vi "EnqueueManualMode.vi"(6 "Priority?":bool, 8 "error in (no error)":errorcluster, 9 "Data":variant, 10 "Message":T1, 11 "queue":refnum<queue>) -> (0 "error out":errorcluster, 3 "queue out":refnum<queue>)   [LabVIEW 2019, in "ManualMode.lvlib"]
uses:
  ManualMode.lvlib
  Enum - ManualModeMessage.ctl
  Cluster - ManualModeMessageCluster.ctl
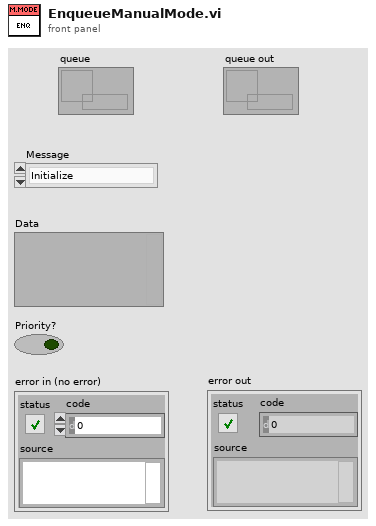
[diagram p1: front panel]
types:
  T1 = typedef "ManualMode.lvlib/Enum - ManualModeMessage.ctl" = enum16{"Initialize", "Idle", "Start", "Stop", "Pause", "Resume", "BroadcastPreCollection", "MoveCCW", "MoveCW", "StopMove", "SetZero", "GotoZero", "UpdateHW", "SendMark10Cmd", "ReadPosition", "ReadTorque", "ReadStatus", "Error", "Exit"}
  T2 = typedef "ManualMode.lvlib/Cluster - ManualModeMessageCluster.ctl" = cluster{"Message":T1, "Data":variant}
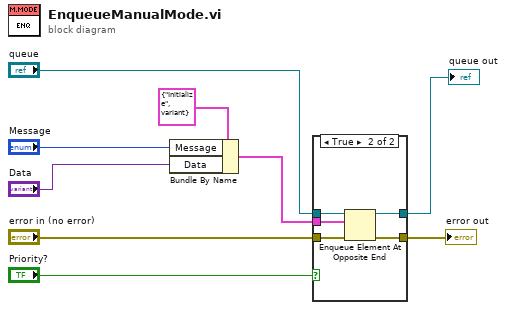
[diagram p0: block diagram]
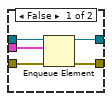
[diagram p2: hidden frame]
diagram:
  n1 = Bundle By Name(cluster=T2 {"Message"=enum."Initialize", "Data"=variant} ("element"), "Message"="Message", "Data"="Data") -> (w7:T2)
  n2 = case shown="True" "Priority?" {
    tunnel: [w14 w18] -> w9
    tunnel: w7 -> [w13 w15]
    tunnel: "queue" -> [w12 w17]
    tunnel: "error in (no error)" -> [w11 w19]
    tunnel: [w10 w16] -> w2
    frame False {
      n3 = Enqueue Element(queue=w12, element=w13, error in (no error)=w11) -> (queue out=w10:refnum<queue>, error out=w14:errorcluster)  [unwired: 1 in, 1 out]
    }
    frame True {
      n4 = Enqueue Element At Opposite End(queue=w17, element=w15, error in (no error)=w19) -> (queue out=w16:refnum<queue>, error out=w18:errorcluster)  [unwired: 1 in, 1 out]
    }
  }
  "error out" <- w9
  "queue out" <- w2
